vi "Pert_MotorSelection.vi"(4 "Pert Direction":i16, 6 "y_Fdesired":dbl, 7 "condition":bool) -> (2 "DesTensions":dbl[](array[numeric]))   [LabVIEW 2017]
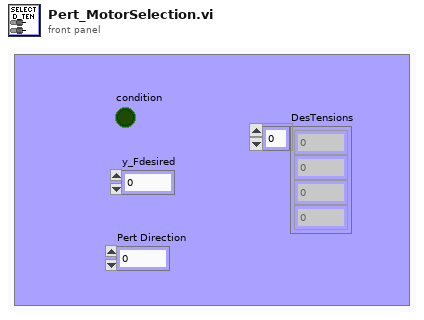
[diagram p1: front panel]
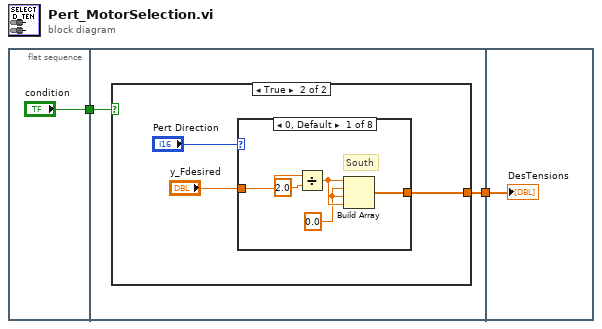
[diagram p0: block diagram]
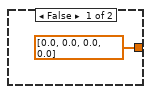
[diagram p2: hidden frame]
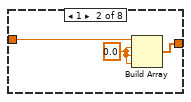
[diagram p3: hidden frame]
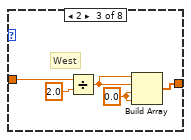
[diagram p4: hidden frame]
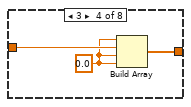
[diagram p5: hidden frame]
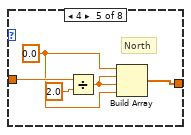
[diagram p6: hidden frame]
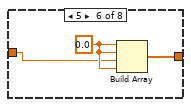
[diagram p7: hidden frame]
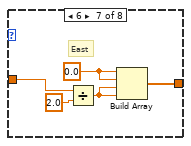
[diagram p8: hidden frame]
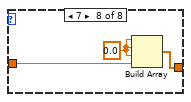
[diagram p9: hidden frame]
diagram:
  n1 = flat-sequence {
    tunnel: ["condition"] -> w2
    tunnel: w2 -> [w5]
    tunnel: [w4] -> w1
    tunnel: w1 -> [w42]
    frame #0 {
    }
    frame #1 {
      n2 = case shown="True" w5 {
        tunnel: [dbl[] [0.0, 0.0, 0.0, 0.0] w7] -> w4
        frame False {
        }
        frame True {
          n3 = case shown="0, Default" "Pert Direction" {
            tunnel: "y_Fdesired" -> [w13 w17 w19 w24 w29 w32 w35 w41]
            tunnel: [w10 w15 w18 w25 w26 w31 w34 w39] -> w7
            frame 0, Default {
              w11 = 0.0 ("element")
              # "South"
              n4 = Divide(x=w13, y=2.0) -> (x/y=w12:dbl)
              n5 = Build Array(w12, w11, w11, w12) -> (w10:dbl[])
            }
            frame 1 {
              w16 = 0.0 ("element")
              n6 = Build Array(w17, w16, w16, w16) -> (w15:dbl[])
            }
            frame 2 {
              w21 = 0.0 ("element")
              # "West"
              n7 = Divide(x=w19, y=2.0) -> (x/y=w20:dbl)
              n8 = Build Array(w20, w20, w21, w21) -> (w18:dbl[])
            }
            frame 3 {
              w23 = 0.0 ("element")
              n9 = Build Array(w23, w24, w23, w23) -> (w25:dbl[])
            }
            frame 4 {
              w27 = 0.0 ("element")
              # "North"
              n10 = Divide(x=w29, y=2.0) -> (x/y=w28:dbl)
              n11 = Build Array(w27, w28, w28, w27) -> (w26:dbl[])
            }
            frame 5 {
              w33 = 0.0 ("element")
              n12 = Build Array(w33, w33, w32, w33) -> (w31:dbl[])
            }
            frame 6 {
              w37 = 0.0 ("element")
              # "East"
              n13 = Divide(x=w35, y=2.0) -> (x/y=w36:dbl)
              n14 = Build Array(w37, w37, w36, w36) -> (w34:dbl[])
            }
            frame 7 {
              w40 = 0.0 ("element")
              n15 = Build Array(w40, w40, w40, w41) -> (w39:dbl[])
            }
          }
        }
      }
    }
    frame #2 {
      "DesTensions" <- w42
    }
  }
